vi "Turret_Execute.vi"() -> ()   [LabVIEW 2019]
uses:
  Turret_Globals.vi
  Globals/Sensor_Values.vi
  Turret_States.ctl
  Utility_VIs/Basic_Motor_Modes.ctl
panel:
  out "Waveform Chart":cluster{"Goal Wheel Position":dbl, dbl}(graph)
  in  "Kp_Degrees":dbl=0.07
  in  "Kd Aim":dbl=0.001
  in  "Ki Aim":dbl=1e-05
  in  "upper_limit(degrees)":dbl=160.0
  in  "lower_limit(degrees)":dbl=-160.0
  out "Turret_Spin_Speed":dbl
  in  "Kp Aim":dbl=0.06
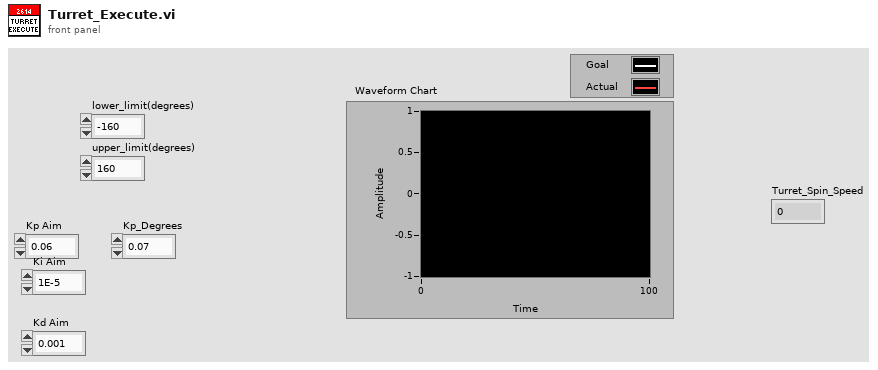
[diagram p1: front panel]
types:
  T1 = typedef "Turret_States.ctl" = enum16{"Manual_Percent_Voltage", "Manual_Speed_Control", "Auto-Target", "Command_TurnToPosition", "Command_Auto_Target", "GoToZero"}
  T2 = typedef "Basic_Motor_Modes.ctl" = enum16{"Percent_Voltage", "Speed_Control", "Position_Control", "Current"}
  T3 = typedef "Turret_Cluster.ctl" = cluster{"Auto-Target?":bool, "Control_State":T1, "Turret_Spin_Speed":dbl, "Turret_Spin_Speed_Control?":bool, "Step":dbl, "Parameter_1":dbl, "Parameter_2":dbl, "Parameter_3":dbl, "Auto_Notifier":refnum<notifier>, "GoToZero?":bool}
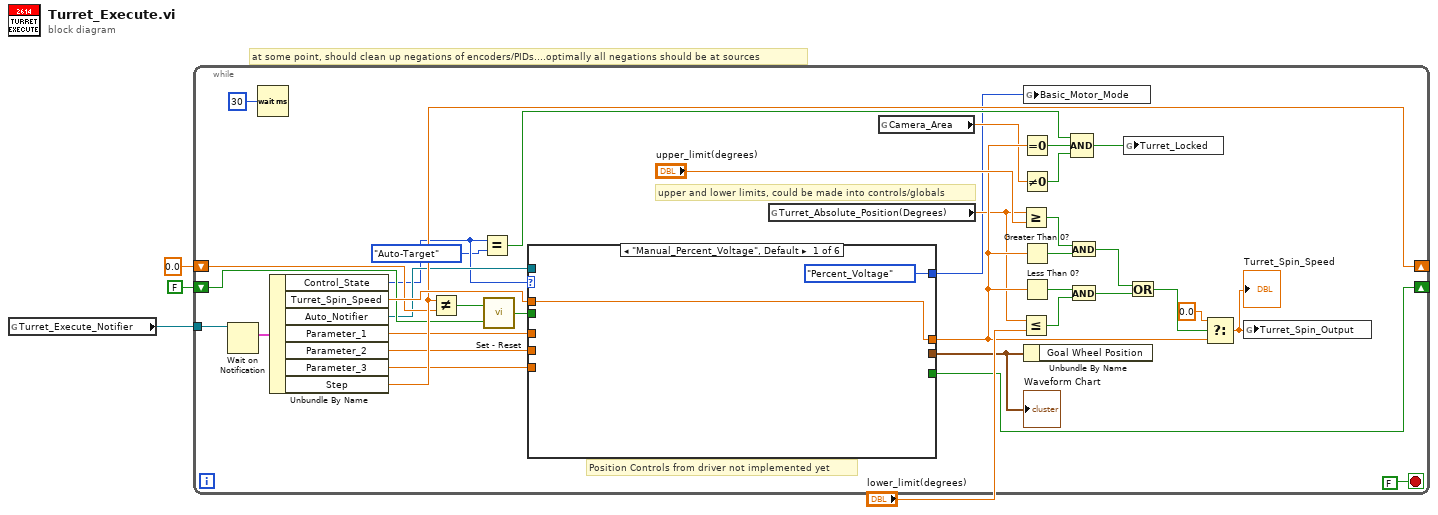
[diagram p0: block diagram]
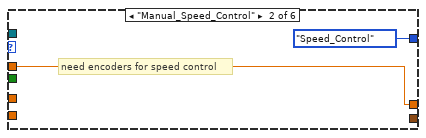
[diagram p2: hidden frame]
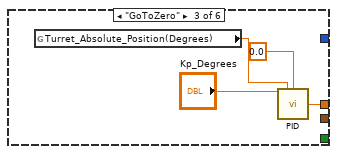
[diagram p3: hidden frame]
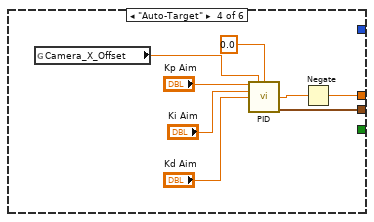
[diagram p4: hidden frame]
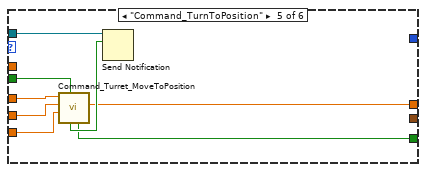
[diagram p5: hidden frame]
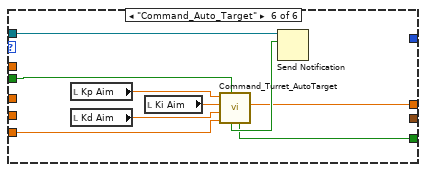
[diagram p6: hidden frame]
diagram:
  # "at some point, should clean up negations of encoders/PIDs....optimally all negations should be at sources"
  n1 = global read "Turret_Globals.vi" "Turret_Execute_Notifier"() -> (w3:refnum<notifier>)
  n2 = while {
    tunnel: w3 -> [w39]
    shift-right: [w25] -> _
    shift-left: 0.0 ("Step") -> [w24]
    shift-right: [w16] -> _
    shift-left: FALSE ("Output") -> [w22]
    stop <- FALSE stop-if-true
    # "Position Controls from driver not implemented yet"
    # "upper and lower limits, could be made into controls/globals"
    n3 = Wait on Notification(notifier=w39) -> (notification=w38:T3)  [unwired: 3 in, 3 out]
    n4 = Wait (ms)(milliseconds to wait=u32 30) -> ()  [unwired: 1 out]
    n5 = Unbundle By Name(w38) -> ("Control_State"=w15:T1, "Turret_Spin_Speed"=w37:dbl, "Auto_Notifier"=w17:refnum<notifier>, "Parameter_1"=w21:dbl, "Parameter_2"=w20:dbl, "Parameter_3"=w19:dbl, "Step"=w25:dbl)
    n6 = Not Equal?(x=w25, y=w24) -> (x != y?=w23:bool)
    n7 = Equal?(x=w15, y=Turret_States."Auto-Target") -> (x = y?=w11:bool)
    n8 = call "Set - Reset.vi"("Reset"=w22, "Set"=w23) -> ("Output"=w18:bool)
    n9 = case shown="\"Manual_Percent_Voltage\", Default" w15 {
      tunnel: w37 -> [w42 w44 _ _ _ _]
      tunnel: [w42 w44 w45 w52 w57 w65] -> w13
      tunnel: w21 -> [_ _ _ _ w64 _]
      tunnel: w20 -> [_ _ _ _ w63 _]
      tunnel: w19 -> [_ _ _ _ w62 w70]
      tunnel: w18 -> [_ _ _ _ w61 w69]
      tunnel: w17 -> [_ _ _ _ w60 w68]
      tunnel: [_ _ _ _ w58 w66] -> w16
      tunnel: [_ _ _ w49 _ _] -> w6
      tunnel: [Basic_Motor_Modes."Percent_Voltage" ("Motor_Mode") Basic_Motor_Modes."Speed_Control" ("Motor_Mode") _ _ _ _] -> w4
      frame "Manual_Percent_Voltage", Default {
      }
      frame "Manual_Speed_Control" {
        # "need encoders for speed control"
      }
      frame "GoToZero" {
        n10 = global read "Sensor_Values.vi" "Turret_Absolute_Position(Degrees)"() -> (w48:dbl)
        n11 = call "PID.vi"("Kp"="Kp_Degrees", "Process Variable"=w48, "Goal"=0.0) -> ("Command"=w45:dbl)  [unwired: 10 in, 2 out]
      }
      frame "Auto-Target" {
        n12 = global read "Sensor_Values.vi" "Camera_X_Offset"() -> (w53:dbl)
        n13 = call "PID.vi"("Kp"="Kp Aim", "Process Variable"=w53, "Goal"=0.0, "Ki"="Ki Aim", "Kd"="Kd Aim") -> ("Command"=w55:dbl, "PID Tracking"=w49:cluster{"Goal Wheel Position":dbl, dbl})  [unwired: 8 in, 1 out]
        n14 = Negate(x=w55) -> (-x=w52:dbl)
      }
      frame "Command_TurnToPosition" {
        n15 = call "Command_Turret_MoveToPosition.vi"("Startup"=w61, "Timeout"=w62, "Speed"=w63, "Goal_Position"=w64) -> ("Turret_Speed"=w57:dbl, "Reint"=w58:bool, "Completed"=w59:bool)  [unwired: 5 in]
        n16 = Send Notification(notification=w59, notifier=w60) -> ()  [unwired: 1 in, 2 out]
      }
      frame "Command_Auto_Target" {
        n17 = local read "Kp Aim"() -> (w73:dbl)
        n18 = local read "Kd Aim"() -> (w71:dbl)
        n19 = local read "Ki Aim"() -> (w72:dbl)
        n20 = call "Command_Turret_AutoTarget.vi"("Startup"=w69, "Timeout"=w70, "Kd"=w71, "Ki"=w72, "Kp"=w73) -> ("Turret_Speed"=w65:dbl, "Reint"=w66:bool, "Completed"=w67:bool)  [unwired: 4 in]
        n21 = Send Notification(notification=w67, notifier=w68) -> ()  [unwired: 1 in, 2 out]
      }
    }
    "Waveform Chart" <- w6
    n22 = global read "Sensor_Values.vi" "Turret_Absolute_Position(Degrees)"() -> (w7:dbl)
    n23 = global read "Sensor_Values.vi" "Camera_Area"() -> (w9:dbl)
    n24 = Greater Or Equal?(x=w7, y="upper_limit(degrees)") -> (x >= y?=w36:bool)
    n25 = Less Or Equal?(x=w7, y="lower_limit(degrees)") -> (x <= y?=w28:bool)
    n26 = Equal To 0?(x=w13) -> (x = 0?=w10:bool)
    n27 = Not Equal To 0?(x=w9) -> (x != 0?=w8:bool)
    n28 = Greater Than 0?(x=w13) -> (x > 0?=w35:bool)
    n29 = Less Than 0?(x=w13) -> (x < 0?=w34:bool)
    n30 = global write "Turret_Globals.vi" "Basic_Motor_Mode"(w4) -> ()
    n31 = Unbundle By Name(w6) -> ()  [unwired: 1 out]
    n32 = And(x=w36, y=w35) -> (x .and. y?=w32:bool)
    n33 = And(x=w34, y=w28) -> (x .and. y?=w33:bool)
    n34 = Compound Arithmetic op=AND(w11, w10, w8) -> (w12:bool)
    n35 = global write "Turret_Globals.vi" "Turret_Locked"(w12) -> ()
    n36 = Or(x=w32, y=w33) -> (x .or. y?=w31:bool)
    n37 = Select(t=0.0, s=w31, f=w13) -> (s? t:f=w5:dbl)
    "Turret_Spin_Speed" <- w5
    n38 = global write "Turret_Globals.vi" "Turret_Spin_Output"(w5) -> ()
  }
